vi "File Manager.vi"(4 "Use Record Time":bool, 5 "Volt Channel":T1={"Index"=[], "Chl Name"=[], "Scale"=[], "Offset"=[], "Sample Rate"=100, "Device Name"="", "Channel"=""}, 6 "Record Time (s)":dbl=10.0, 7 "Enum":T2=enum."Close File", 8 "error in":errorcluster, 9 "Voltage":waveform(dbl)[](array[waveform]), 10 "File Choice":T3, 11 "File Name":string) -> (0 "error out":errorcluster, 1 "Recording":bool, 2 "timeout":i32, 3 "File Path":path)   [LabVIEW 2021]
doc: "This vi has four functions:\nCreate File - Create a new TDMS or CSV file depending on user choice. If user filled in file name, use that file name with time infomation. If user didn't filled in file name, use \"Experiment Result \"+time information.\nConfig Data - Save Channel Number, Channel Name, Scale and Offset into file.\nVolt Data - Create Time array and merge with Voltage Data, then save them into file. \nClost File - Close file and reset all parameters."
uses:
  Control/File Choice Enum.ctl
  Control/File Manager Enum.ctl
  Control/Volt Chl.ctl
  File Abstract Class/File Abstract.lvclass
  TDMS File Class/TDMS File.lvclass
  CSV File Class/CSV File.lvclass
  Control/File Information Cluster.ctl
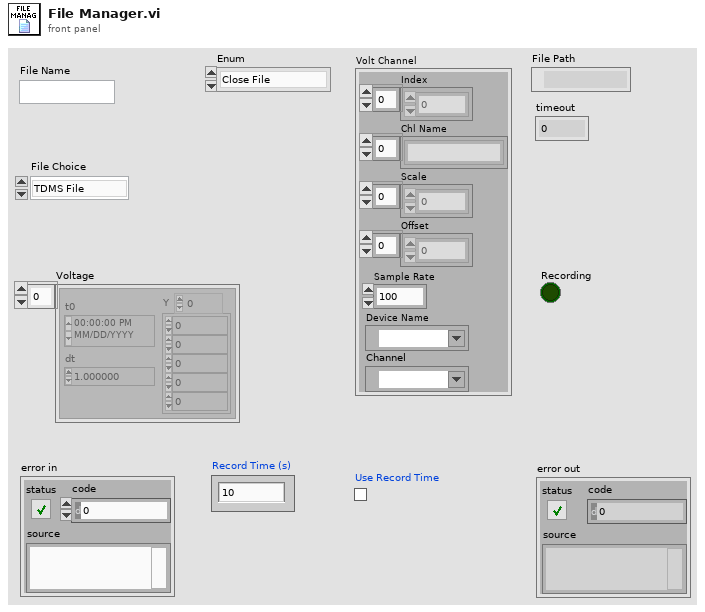
[diagram p1: front panel]
types:
  T1 = typedef "Volt Chl.ctl" = cluster{"Index":i32[], "Chl Name":string[], "Scale":dbl[], "Offset":dbl[], "Sample Rate":i32, "Device Name":tag, "Channel":tag}
  T2 = typedef "File Manager Enum.ctl" = enum16{"Create File", "Config Data", "Volt Data", "Close File"}
  T3 = typedef "File Choice Enum.ctl" = enum16{"TDMS File", "CSV File"}
  T4 = typedef "File Information Cluster.ctl" = cluster{"File Refnum":variant, "Chl Name":string[]}
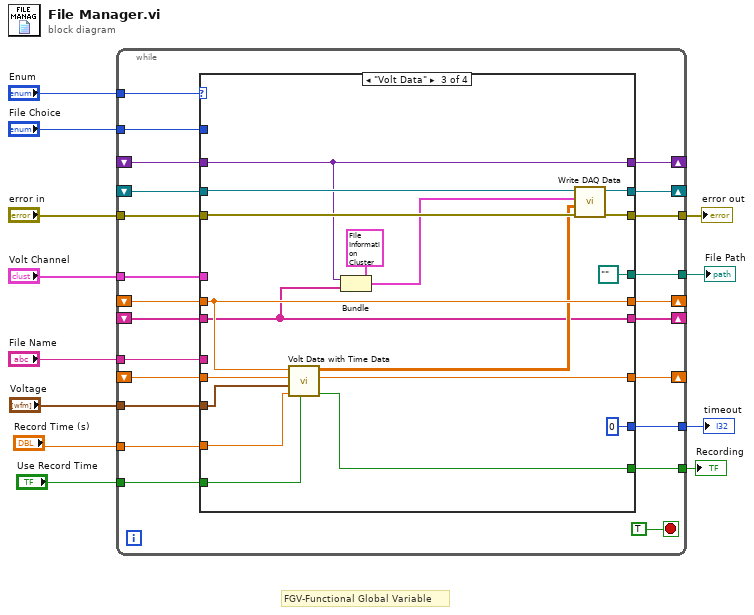
[diagram p0: block diagram]
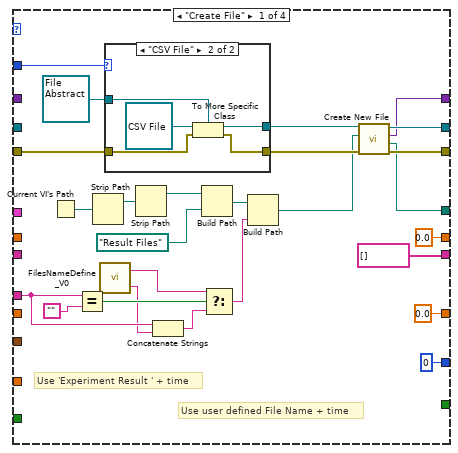
[diagram p2: hidden frame]
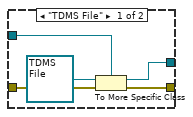
[diagram p3: hidden frame]
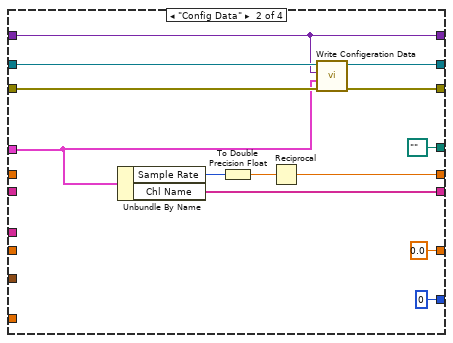
[diagram p4: hidden frame]
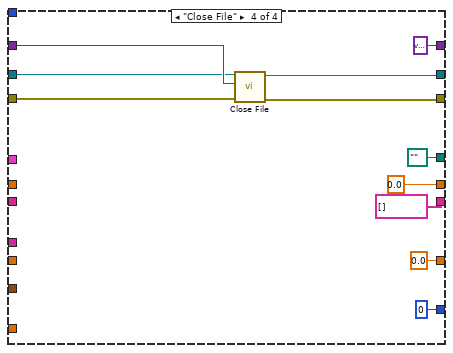
[diagram p5: hidden frame]
diagram:
  # "FGV-Functional Global Variable"
  n1 = while {
    tunnel: "File Name" -> [w35]
    tunnel: "File Choice" -> [w34]
    tunnel: [w31] -> w10
    shift-right: [w32] -> _
    shift-left: _ -> [w28]
    tunnel: "error in" -> [w30]
    tunnel: "Enum" -> [w29]
    tunnel: "Volt Channel" -> [w27]
    shift-right: [w26] -> _
    shift-left: _ -> [w25]
    tunnel: [w24] -> w6
    shift-right: [w23] -> _
    shift-left: _ -> [w22]
    shift-right: [w21] -> _
    shift-left: _ -> [w20]
    shift-right: [w19] -> _
    shift-left: _ -> [w18]
    tunnel: "Voltage" -> [w17]
    tunnel: "Record Time (s)" -> [w16]
    tunnel: [w15] -> w3
    tunnel: "Use Record Time" -> [w14]
    tunnel: [w13] -> w1
    stop <- TRUE stop-if-true
    n2 = case shown="\"Volt Data\"" w29 {
      tunnel: w35 -> [w38 _ _ _]
      tunnel: w34 -> [w56 _ _ _]
      tunnel: [w55 w83 w99 w109] -> w32
      tunnel: [w54 w82 w100 w110] -> w31
      tunnel: w30 -> [w53 w81 w101 w111]
      tunnel: w28 -> [_ w84 w102 w112]
      tunnel: w27 -> [_ w78 _ _]
      tunnel: [w52 w80 w96 variant ("File Refnum")] -> w26
      tunnel: w25 -> [_ w80 w96 w113]
      tunnel: [w44 path "" ("appended path") path "" ("appended path") path "" ("appended path")] -> w24
      tunnel: [0.0 w75 w94 0.0] -> w23
      tunnel: w22 -> [_ _ w94 _]
      tunnel: [string[] [] ("Chl Name") w74 w91 string[] [] ("Chl Name")] -> w21
      tunnel: w20 -> [_ _ w91 _]
      tunnel: [0.0 0.0 w89 0.0 ("t_start out")] -> w19
      tunnel: w18 -> [_ _ w90 _]
      tunnel: w17 -> [_ _ w93 _]
      tunnel: w16 -> [_ _ w88 _]
      tunnel: [0 ("timeout") 0 ("timeout") 0 ("timeout") 0 ("timeout")] -> w15
      tunnel: w14 -> [_ _ w87 _]
      tunnel: [_ _ w86 _] -> w13
      frame "Create File" {
        # "Use 'Experiment Result ' + time"
        # "Use user defined File Name + time"
        n3 = Current VI's Path() -> (path=w60:path)
        n4 = Equal?(x=w38, y="") -> (x = y?=w47:bool)
        n5 = Strip Path(path=w60) -> (stripped path=w61:path)  [unwired: 1 out]
        n6 = call "FilesNameDefine_V0.vi"() -> ("date/time string"=w37:string, "Result File Name"=w39:string)  [unwired: 2 in]
        n7 = case shown="\"CSV File\"" w56 {
          tunnel: refnum<class "File Abstract.lvclass"> refnum ("File Manager.lvclass") -> [w65 w71]
          tunnel: [w63 w69] -> w58
          tunnel: [w64 w68] -> w59
          tunnel: w53 -> [w62 w67]
          frame "TDMS File" {
            n8 = To More Specific Class(target class=w65, reference=refnum<class "TDMS File.lvclass"> refnum ("TDMS File.lvclass"), error in=w62) -> (specific class reference=w64:refnum<class "File Abstract.lvclass">, error out=w63:errorcluster)
          }
          frame "CSV File" {
            n9 = To More Specific Class(target class=w71, reference=refnum<class "CSV File.lvclass"> refnum ("CSV File.lvclass"), error in=w67) -> (specific class reference=w68:refnum<class "File Abstract.lvclass">, error out=w69:errorcluster)
          }
        }
        n10 = Strip Path(path=w61) -> (stripped path=w51:path)  [unwired: 1 out]
        n11 = Concatenate Strings(w38, w37) -> (w36:string)
        n12 = Build Path(base path=w51, name or relative path=path "Result Files") -> (appended path=w50:path)
        n13 = Select(t=w39, s=w47, f=w36) -> (s? t:f=w46:string)
        n14 = Build Path(base path=w50, name or relative path=w46) -> (appended path=w45:path)
        n15 = call-dynamic "Create New File.vi"("error in (no error)"=w58, "Path"=w45, "File Manager in"=w59) -> ("error out"=w54:errorcluster, "Path out"=w44:path, "File Refnum"=w52:variant, "File Manager out"=w55:refnum<class "File Abstract.lvclass">)  [unwired: 5 in]
      }
      frame "Config Data" {
        n16 = Unbundle By Name(w78) -> ("Sample Rate"=w77:i32, "Chl Name"=w74:string[])
        n17 = To Double Precision Float(number=w77) -> (double precision float=w76:dbl)
        n18 = Reciprocal(x=w76) -> (1/x=w75:dbl)
        n19 = call-dynamic "Write Configeration Data.vi"("error in (no error)"=w81, "Volt Channel"=w78, "File Refnum"=w80, "File Manager in"=w84) -> ("error out"=w82:errorcluster, "File Manager out"=w83:refnum<class "File Abstract.lvclass">)  [unwired: 6 in]
      }
      frame "Volt Data" {
        n20 = call "Volt Data with Time Data.vi"("Use Record Time"=w87, "Record Time (s)"=w88, "Voltage"=w93, "t_start in"=w90, "dt"=w94) -> ("Recording"=w86:bool, "t_start out"=w89:dbl, "Data with Time"=w92:dbl[][])  [unwired: 3 in, 1 out]
        n21 = Bundle(cluster=T4 {"File Refnum"=variant, "Chl Name"=[]} ("File Infor"), "File Refnum"=w96, "Chl Name"=w91) -> (w97:T4)
        n22 = call-dynamic "Write DAQ Data.vi"("error in (no error)"=w101, "Voltage with Time"=w92, "File Infor"=w97, "File Manager in"=w102) -> ("error out"=w100:errorcluster, "File Manager out"=w99:refnum<class "File Abstract.lvclass">)  [unwired: 6 in]
      }
      frame "Close File" {
        n23 = call-dynamic "Close File.vi"("error in (no error)"=w111, "File Refnum"=w113, "File Manager in"=w112) -> ("error out"=w110:errorcluster, "File Manager out"=w109:refnum<class "File Abstract.lvclass">)  [unwired: 7 in]
      }
    }
  }
  "error out" <- w10
  "File Path" <- w6
  "timeout" <- w3
  "Recording" <- w1
